vi "Open.vi"(8 "error in (no error)":errorcluster, 9 "Open FP? (F)":bool, 10 "Server Title":string, 11 "Server Port in":u16) -> (0 "error out":errorcluster, 2 "Http Server":string, 3 "Server Port out":u16)   [LabVIEW 2021, in "HttpServer.lvlib"]
uses:
  HttpServer.lvlib
  TypeDefs/Action.ctl
  SubVIs/Tcp Daemon.vi
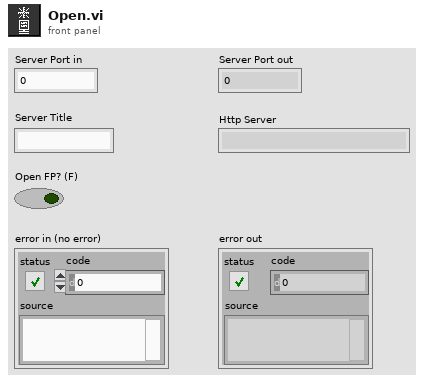
[diagram p1: front panel]
types:
  T1 = typedef "HttpServer.lvlib/Action.ctl" = enum8{"noop", "add", "get", "set", "remove"}
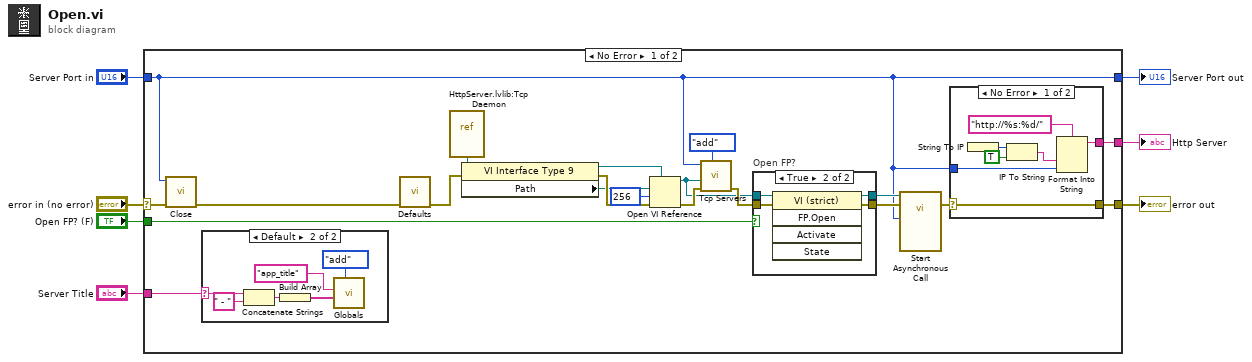
[diagram p0: block diagram]
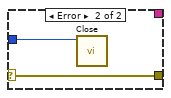
[diagram p4: hidden frame]
diagram:
  n1 = case shown="No Error" "error in (no error)" {
    selector: "error in (no error)" -> [w15 w50]
    tunnel: "Server Port in" -> [w13 w49]
    tunnel: [w14 w50] -> w5
    tunnel: [w13 w49] -> w4
    tunnel: "Open FP? (F)" -> [w12 _]
    tunnel: [w9 _] -> w2
    tunnel: "Server Title" -> [w8 _]
    frame No Error {
      n2 = call "Close.vi"("error in (no error)"=w15, "Server Port in"=w13) -> ("error out"=w11:errorcluster)  [unwired: 8 in, 1 out]
      n3 = case shown="Default" w8 {
        selector: w8 -> [_ w32]
        frame "" {
        }
        frame Default {
          n4 = Concatenate Strings(w32, " - " ("string")) -> (w29:string)
          n5 = Build Array(w29) -> (w31:string[])
          n6 = call "Globals.vi"("Action"=Action."add", "Values in"=w31, "Key"="app_title") -> ()  [unwired: 5 in, 4 out]
        }
      }
      n7 = call "Defaults.vi"("error in (no error)"=w11) -> ("error out"=w10:errorcluster)  [unwired: 10 in]
      n8 = vi-ref "HttpServer.lvlib:Tcp Daemon.vi"() -> (w23:refnum<vi>)
      n9 = property class="VI Interface Type 9"(reference=w23, error in=w10) -> (reference out=w22:refnum<vi>, error out=w26:errorcluster, "Path"=w25:path)
      n10 = Open VI Reference(type specifier VI Refnum (for type only)=w22, vi path=w25, options=256, error in (no error)=w26) -> (vi reference=w16:refnum<vi>, error out=w18:errorcluster)  [unwired: 2 in]
      n11 = call "Tcp Servers.vi"("Action"=Action."add", "error in (no error)"=w18, "VI in"=w16, "Server Port in"=w13) -> ("error out"=w17:errorcluster)  [unwired: 4 in, 3 out]
      n12 = case "Open FP?" shown="True" w12 {
        tunnel: [w35 w39] -> w20
        tunnel: [w34 w38] -> w19
        tunnel: w17 -> [w35 w37]
        tunnel: w16 -> [w34 w36]
        frame False {
        }
        frame True {
          n13 = invoke class="VI (strict)" method="FP.Open"(reference=w36, error in=w37) -> (reference out=w38:refnum<vi>, error out=w39:errorcluster)  [unwired: 3 in, 3 out]
        }
      }
      n14 = call-by-ref "Start Asynchronous Call"(reference=w19, error in=w20, "Http Port"=w13) -> (error out=w21:errorcluster)  [unwired: 11 in, 1 out]
      n15 = case shown="No Error" w21 {
        selector: w21 -> [w46 w47]
        tunnel: w13 -> [w45 w48]
        tunnel: [w46 w47] -> w14
        tunnel: [w40 _] -> w9
        frame No Error {
          n16 = String To IP() -> (0:w44:u32)  [unwired: 1 in]
          n17 = IP To String(1:TRUE ("dot notation? (F)"), 2:w44) -> (0:w42:string)
          n18 = Format Into String(format string="http://%s:%d/", w42, w45) -> (resulting string=w40:string)  [unwired: 2 in, 1 out]
        }
        frame Error {
          n19 = call "Close.vi"("Server Port in"=w48) -> ()  [unwired: 9 in, 2 out]
        }
      }
    }
    frame Error {
    }
  }
  "error out" <- w5
  "Server Port out" <- w4
  "Http Server" <- w2
